vi "c SIM Spark Restore Factory Defaults.vi"(8 "error in (no error)":errorcluster, 9 "resetAll":bool, 10 "persist":bool, 11 "handle":T1) -> (0 "error out":errorcluster, 2 "function return":T2, 3 "handle out":T1)   [LabVIEW 2023, in "REVLibDriver.lvlib"]
doc: "c_REVLib_ErrorCode c_SIM_Spark_RestoreFactoryDefaults(c_SIM_Spark_handle handle,\n bool persist,\n bool resetAll);"
uses:
  REVLibDriver.lvlib
  REVLibDriver.dll
  Custom Controls/c_Spark_handle.ctl
  subvi/RevLibError.ctl
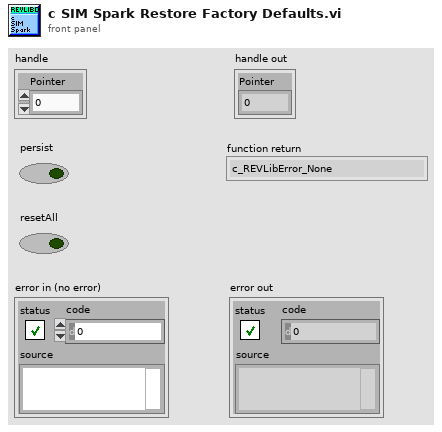
[diagram p1: front panel]
types:
  T1 = typedef "REVLibDriver.lvlib/c_Spark_handle.ctl" = cluster{"Pointer":u64}
  T2 = typedef "REVLibDriver.lvlib/RevLibError.ctl" = enum16{"c_REVLibError_None", "c_REVLibError_General", "c_REVLibError_CANTimeout", "c_REVLibError_NotImplemented", "c_REVLibError_HAL", "c_REVLibError_CantFindFirmware", "c_REVLibError_FirmwareTooOld", "c_REVLibError_FirmwareTooNew", "c_REVLibError_ParamInvalidID", "c_REVLibError_ParamMismatchType", "c_REVLibError_ParamAccessMode", "c_REVLibError_ParamInvalid", "c_REVLibError_ParamNotImplementedDeprecated", "c_REVLibError_FollowConfigMismatch", "c_REVLibError_Invalid", "c_REVLibError_SetpointOutOfRange", "c_REVLibError_Unknown", "c_REVLibError_CANDisconnected", "c_REVLibError_DuplicateCANId", "c_REVLibError_InvalidCANId", "c_REVLibError_SparkMaxDataPortAlreadyConfiguredDifferently", "c_REVLibError_SparkFlexBrushedWithoutDock", "c_REVLibError_InvalidBrushlessEncoderConfiguration", "c_REVLibError_FeedbackSensorIncompatibleWithDataPortConfig", "c_REVLibError_ParamInvalidChannel", "c_REVLibError_ParamInvalidValue", "c_REVLibError_CannotPersistParametersWhileEnabled", "c_REVLibError_NotReadyToReceiveCommand", "c_REVLibError_NumCodes"}
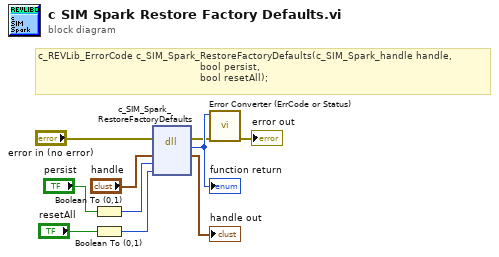
[diagram p0: block diagram]
diagram:
  # "c_REVLib_ErrorCode c_SIM_Spark_RestoreFactoryDefaults(c_SIM_Spark_handle handle,\n                                                      bool persist,\n                                                      bool resetAll);"
  n1 = Boolean To (0,1)(Boolean="persist") -> (0, 1=w6:i16)
  n2 = Boolean To (0,1)(Boolean="resetAll") -> (0, 1=w4:i16)
  n3 = dll-call lib="REVLibDriver.*" fn="c_SIM_Spark_RestoreFactoryDefaults"(error in="error in (no error)", "handle"="handle", "persist"=w6, "resetAll"=w4) -> (error out=w2:errorcluster, w10:u32, "handle"=→"handle out":T1)  [unwired: 4 in, 1 out]
  "function return" <- w10
  n4 = call "Error Converter (ErrCode or Status).vi"("error in (no error)"=w2, "error code"=w10) -> ("error out"=→"error out":errorcluster)  [unwired: 9 in]
